vi "Handle setConfiguration.vi"(8 "error in (no error)":errorcluster, 10 "setConfiguration":variant, 11 "Instrument.Template in":refnum<class "Instrument.LN2.lvclass">) -> (0 "error out":errorcluster, 3 "Instrument.Template out":refnum<class "Instrument.LN2.lvclass">)   [LabVIEW 2019, in "Instrument.LN2.lvclass"]
uses:
  Instrument.LN2.lvclass
  45e4b271-6884-462c-ad3a-d505ab08eb62.vi
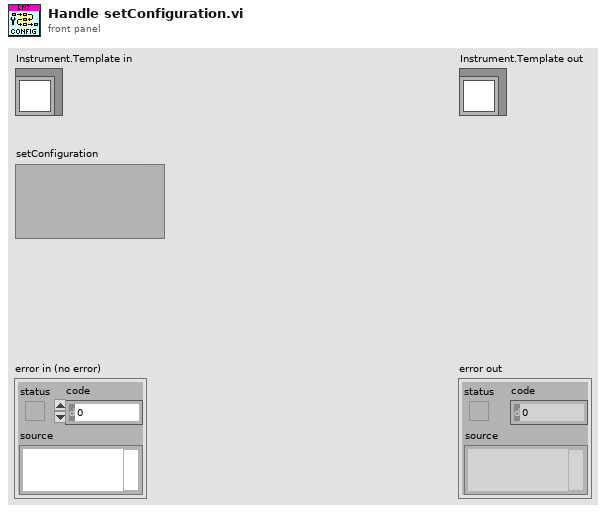
[diagram p1: front panel]
types:
  T1 = typedef "Instrument.LN2.lvclass/Instrument.LN2.Configuration--Cluster.ctl" = cluster{"Example Setting 1":dbl, "Example Setting 2":dbl, "Example Setting 3":string}
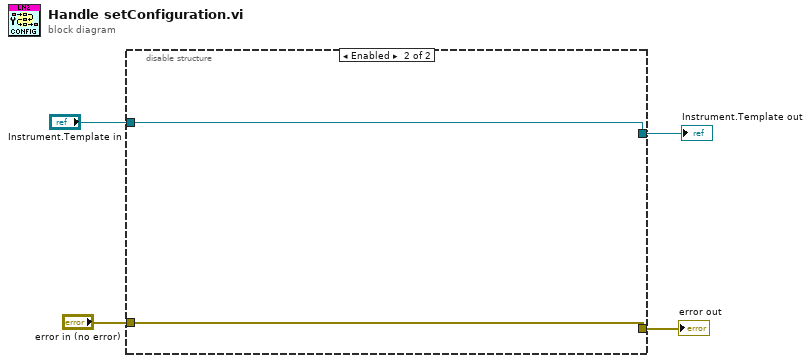
[diagram p0: block diagram]
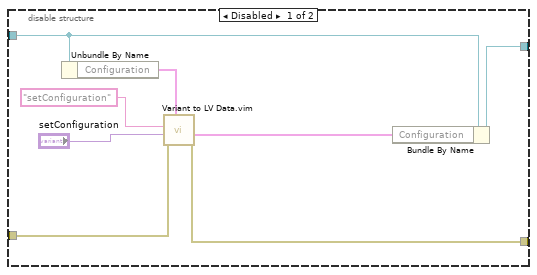
[diagram p2: hidden frame]
diagram:
  n1 = disable-structure shown="Enabled" {
    disable-tunnel: "error in (no error)" -> [w10 w13]
    disable-tunnel: [w9 w13] -> w3
    disable-tunnel: "Instrument.Template in" -> [w7 w14]
    disable-tunnel: [w6 w14] -> w1
    frame Disabled {
      n2 = Unbundle By Name(w7) -> ("Configuration"=w11:T1)
      n3 = call "Variant to LV Data.vim"("type"=w11, "error in (no error)"=w10, "JSON Data in"="setConfiguration", "Command"="setConfiguration") -> ("error out"=w9:errorcluster, "Data out"=w5:T1)  [unwired: 4 in, 2 out]
      n4 = Bundle By Name(cluster=w7, "Configuration"=w5) -> (w6:refnum<class "Instrument.LN2.lvclass">)
    }
    frame Enabled {
    }
  }
  "error out" <- w3
  "Instrument.Template out" <- w1
